vi "Substitute Actor.vi"(10 "Substitute Actor in":refnum<class "Actor.lvclass">, 11 "Current Command Processor":refnum<class "Command Processor Actor.lvclass">) -> (0 "error out":errorcluster, 2 "Substitute Actor out":refnum<class "Actor.lvclass">)   [LabVIEW 2014, in "Robot Actor Framework.lvlib" / "Command Processor Actor.lvlib" / "Command Processor Actor.lvclass"]
doc: "(<B>Filename</B>: Actor Framework.lvlib:Actor.lvclass:Substitute Actor.vi)\n\nThis method copies information from the <b>Current Actor</b> to the <b>Substitute Actor</b>, including the to-self and the to-caller queue references. The purpose of this function is to allow an actor to define a method that replaces itself with another actor, useful for implementing a State Pattern Actor. Child classes should override this method to copy any additional fields that they need from the current to the substitute.\n\nThis method may return error code 678010: Illegal substitution. Overrides of this method may choose to return this error if the new actor is not one that is an appropriate substitute for the current actor, for whatever standards of \"appropriate\" are chosen for the current actor. If returning an error, override VIs should return the unmodified <b>Current Actor</b> as <b>Substitute Actor out</b>."
uses:
  Command Processor Actor.lvclass
  <vilib>/ActorFramework/Actor/Actor.lvclass
  Command Processor Actor.lvclass/Command Processor Actor.ctl
  <vilib>/ni/Actors/State Actor/State Actor/State Actor.lvclass
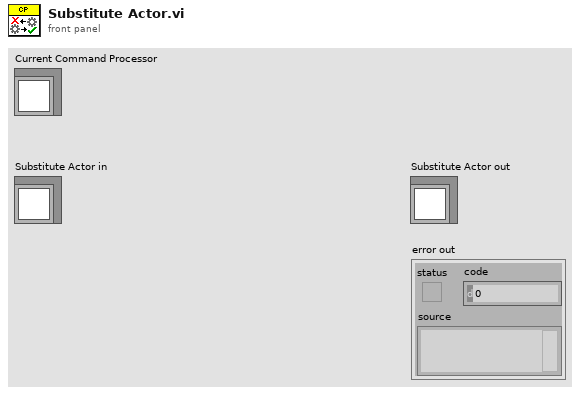
[diagram p1: front panel]
types:
  T1 = typedef "Robot Actor Framework.lvlib/Command Processor Actor.lvlib/Command Processor Actor.lvclass/Command Processor States.ctl" = enum16{"Unknown", "No Command", "Running Command", "Starting Command", "Stopping Command", "Finishing Command"}
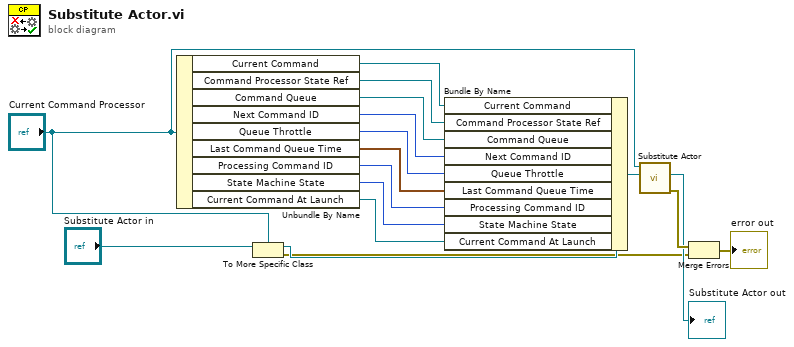
[diagram p0: block diagram]
diagram:
  n1 = Unbundle By Name("Current Command Processor") -> ("Current Command"=w11:refnum<class "Message Enqueuer.lvclass">, "Command Processor State Ref"=w8:refnum<vi>, "Command Queue"=w7:refnum<queue>, "Next Command ID"=w6:u32, "Queue Throttle"=w5:u32, "Last Command Queue Time"=w4:timestamp, "Processing Command ID"=w3:u32, "State Machine State"=w2:T1, "Current Command At Launch"=w1:refnum<class "Command Actor.lvclass">)
  n2 = To More Specific Class(target class="Current Command Processor", reference="Substitute Actor in") -> (specific class reference=w13:refnum<class "Command Processor Actor.lvclass">, error out=w9:errorcluster)  [unwired: 1 in]
  n3 = Bundle By Name(cluster=w13, "Current Command"=w11, "Command Processor State Ref"=w8, "Command Queue"=w7, "Next Command ID"=w6, "Queue Throttle"=w5, "Last Command Queue Time"=w4, "Processing Command ID"=w3, "State Machine State"=w2, "Current Command At Launch"=w1) -> (w12:refnum<class "Command Processor Actor.lvclass">)
  n4 = call-parent "Substitute Actor.vi"("Substitute Actor in"=w12, "Current Actor"="Current Command Processor") -> ("error out"=w17:errorcluster, "Substitute Actor out"=→"Substitute Actor out":refnum<class "Actor.lvclass">)  [unwired: 8 in]
  n5 = Merge Errors(w17, w9) -> (→"error out":errorcluster)
